vi "Generate Column Names.vi"(11 "MeasData":T1) -> (3 "Names (Array)":string[](array[string]), 5 "comma_deli_string":string, 7 "Data":string[][](array[string]))   [LabVIEW 2019]
doc: "Developed by Kevin Thompson\nkevin@thompsonengineering.net\n\nCopyright 2020\nThompson Engineering, LLC"
uses:
  Common/DataQ_SE/TD MeasData--cluster.ctl
  Common/DataTypes/InverterPhaseData--cluster.ctl
panel:
  out "Numeric":i32
  out "Array":variant[](array[variant])
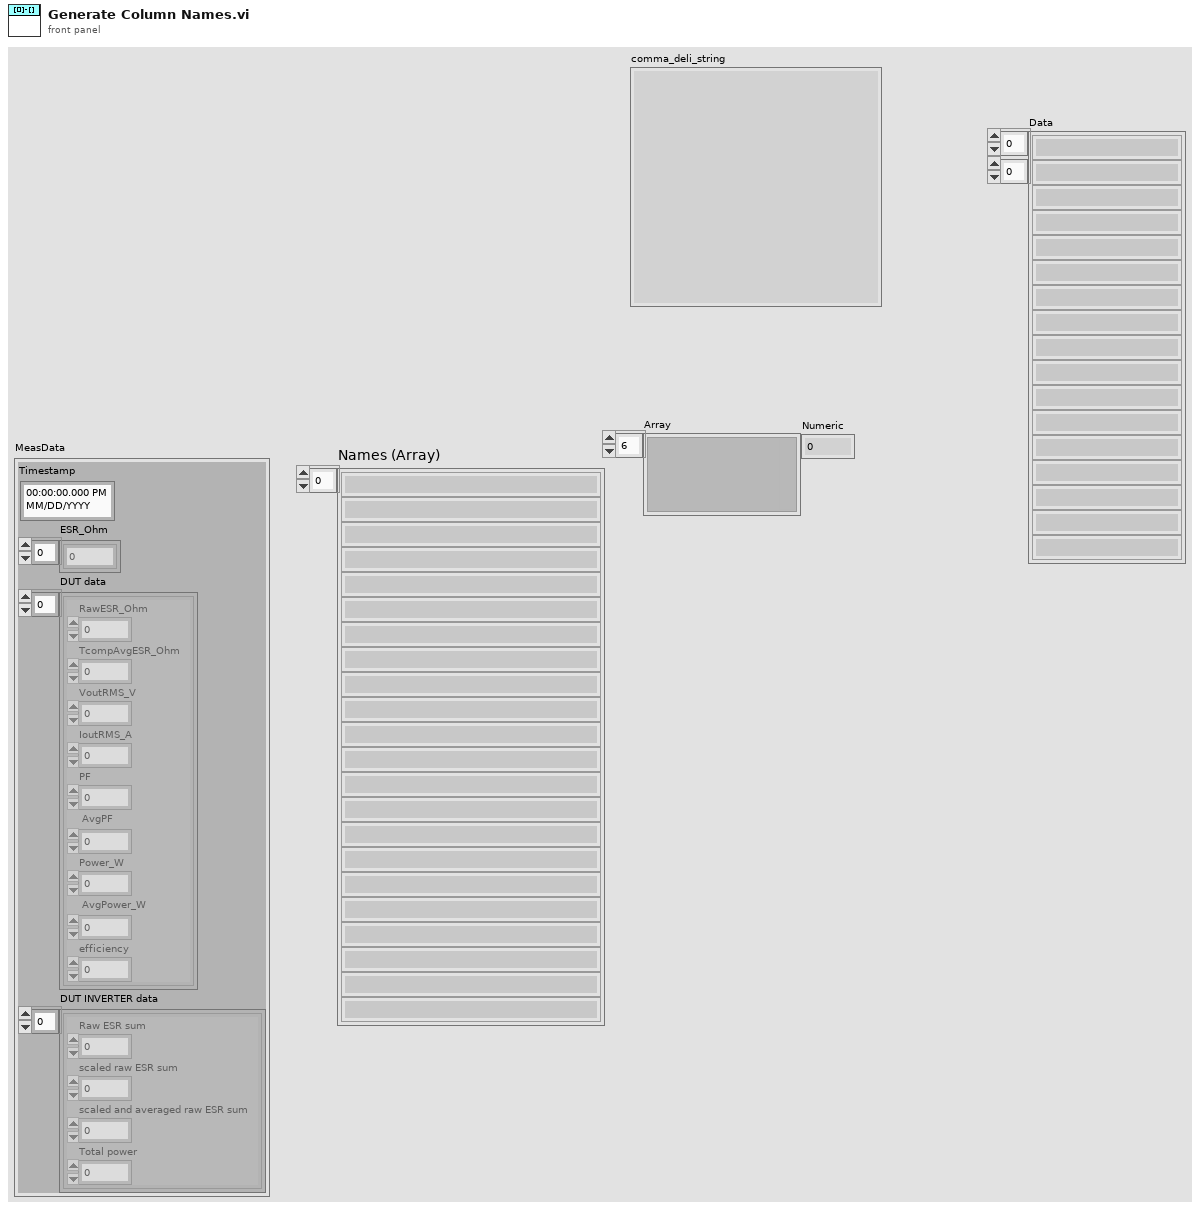
[diagram p1: front panel]
types:
  T1 = typedef "TD MeasData--cluster.ctl" = cluster{"Timestamp":timestamp, "ESR_Ohm":dbl[], "DUT data":T2[], "DUT INVERTER data":cluster{"Raw ESR sum":dbl, "scaled raw ESR sum":dbl, "scaled and averaged raw ESR sum":dbl, "Total power":dbl}[]}
  T2 = typedef "InverterPhaseData--cluster.ctl" = cluster{"RawESR_Ohm":dbl, "TcompAvgESR_Ohm":dbl, "VoutRMS_V":dbl, "IoutRMS_A":dbl, "PF":dbl, "AvgPF":dbl, "Power_W":dbl, "AvgPower_W":dbl, "efficiency":dbl}
  T3 = cluster{"Timestamp":timestamp, "ESR_Ohm":dbl, "Data":T2, "INVERTER data":cluster{"Raw ESR sum":dbl, "scaled raw ESR sum":dbl, "scaled and averaged raw ESR sum":dbl, "Total power":dbl}}
  T4 = cluster{"Raw ESR sum":dbl, "scaled raw ESR sum":dbl, "scaled and averaged raw ESR sum":dbl, "Total power":dbl}[]
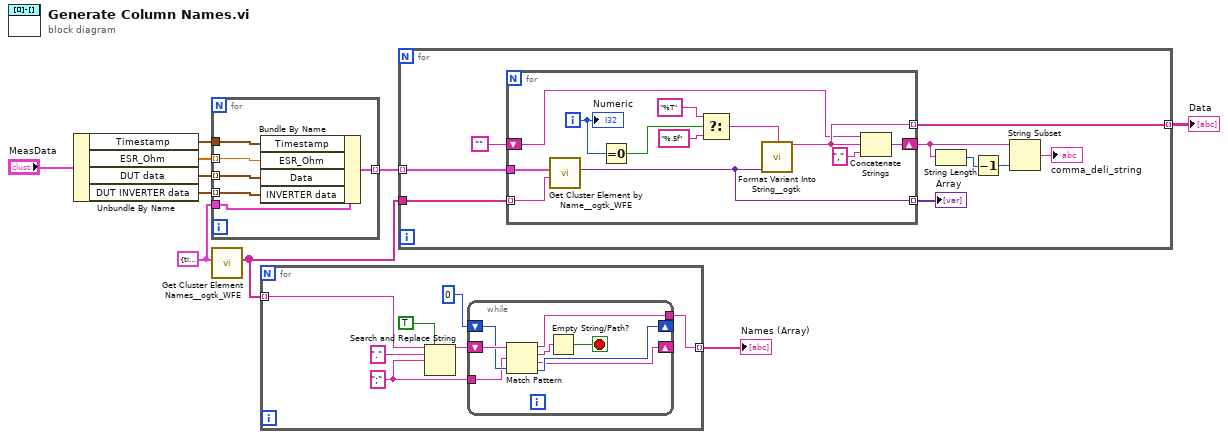
[diagram p0: block diagram]
diagram:
  w4 = T3 {"Timestamp"=timestamp(0 s since 1904-01-01), "ESR_Ohm"=0.0, "Data"={"RawESR_Ohm"=0.0, "TcompAvgESR_Ohm"=0.0, "VoutRMS_V"=0.0, "IoutRMS_A"=0.0, "PF"=0.0, "AvgPF"=0.0, "Power_W"=0.0, "AvgPower_W"=0.0, "efficiency"=0.0}, "INVERTER data"={"Raw ESR sum"=0.0, "scaled raw ESR sum"=0.0, "scaled and averaged raw ESR sum"=0.0, "Total power"=0.0}} ("output cluster")
  n1 = Unbundle By Name("MeasData") -> ("Timestamp"=w8:timestamp, "ESR_Ohm"=w7:dbl[], "DUT data"=w6:T2[], "DUT INVERTER data"=w5:T4)
  n2 = for {
    tunnel: w8 -> [w16]
    tunnel: w7 -> [w15] mode=indexing
    tunnel: w6 -> [w14] mode=indexing
    tunnel: w5 -> [w13] mode=indexing
    tunnel: [w12] -> w2 mode=indexing
    tunnel: w4 -> [w11]
    n3 = Bundle By Name(cluster=w11, "Timestamp"=w16, "ESR_Ohm"=w15, "Data"=w14, "INVERTER data"=w13) -> (w12:T3)
  }
  n4 = call "Get Cluster Element Names__ogtk_WFE.vi"("Variant"=w4) -> ("Names (Array)"=w10:string[])  [unwired: 9 in, 1 out]
  n5 = for {
    tunnel: w10 -> [w22] mode=indexing
    tunnel: [w17] -> w1 mode=indexing
    w18 = ";" ("regular expression")
    n6 = Search and Replace String(replace all?=TRUE ("replace all? (F)"), input string=w22, search string="." ("regular expression"), replace string=w18) -> (result string=w20:string)  [unwired: 4 in, 3 out]
    n7 = while {
      shift-right: [w26] -> _
      shift-left: w20 -> [w31]
      shift-right: [w29] -> _
      shift-left: 0 ("offset past match") -> [w28]
      tunnel: w18 -> [w27]
      tunnel: [w25] -> w17
      stop <- w30 stop-if-true
      n8 = Match Pattern(string=w31, regular expression=w27, offset (0)=w28) -> (before substring=w25:string, match substring=w24:string, after substring=w26:string, offset past match=w29:i32)
      n9 = Empty String/Path?(string/path=w24) -> (empty?=w30:bool)
    }
  }
  "Names (Array)" <- w1
  n10 = for {
    tunnel: w10 -> [w40]
    tunnel: w2 -> [w33] mode=indexing
    tunnel: [w32] -> w3 mode=indexing
    n11 = for {
      tunnel: w33 -> [w43]
      tunnel: w40 -> [w42] mode=indexing
      tunnel: [w41] -> w39 mode=indexing
      tunnel: [w47] -> w32 mode=indexing
      shift-right: [w46] -> w38
      shift-left: "" -> [w44]
      i -> [w52]
      n12 = call "Get Cluster Element by Name__ogtk_WFE.vi"("Element Name"=w42, "Cluster"=w43) -> ("VElement"=w41:variant)  [unwired: 7 in, 2 out]
      n13 = Equal To 0?(x=w52) -> (x = 0?=w51:bool)
      n14 = Select(t="%T" ("Format String"), s=w51, f="%.5f" ("Format String")) -> (s? t:f=w48:string)
      n15 = call <userlib>:"Format Variant Into String__ogtk.vi"("Format String"=w48, "Variant"=w41) -> ("Output String"=w47:string)  [unwired: 12 in, 1 out]
      n16 = Concatenate Strings(w44, w47, ",") -> (w46:string)
      "Numeric" <- w52
    }
    "Array" <- w39
    n17 = String Length(string=w38) -> (length=w37:i32)
    n18 = Decrement(x=w37) -> (x-1=w36:i32)
    n19 = String Subset(string=w38, length (rest)=w36) -> (substring=→"comma_deli_string":string)  [unwired: 1 in]
  }
  "Data" <- w3
